vi "zs_example.vi"() -> ()   [LabVIEW 2014, in "Dialogue.lvlib" / "Dialogue.lvclass"]
uses:
  Dialogue.lvclass
  ctl/Point.ctl
panel:
  out "数值":dbl
  out "机器人语音指令数据簇数组(Voice)":T1(array[cluster])
  out "连接的字符串 2":string
  out "连接的字符串":string
  out "值(信号)":T2
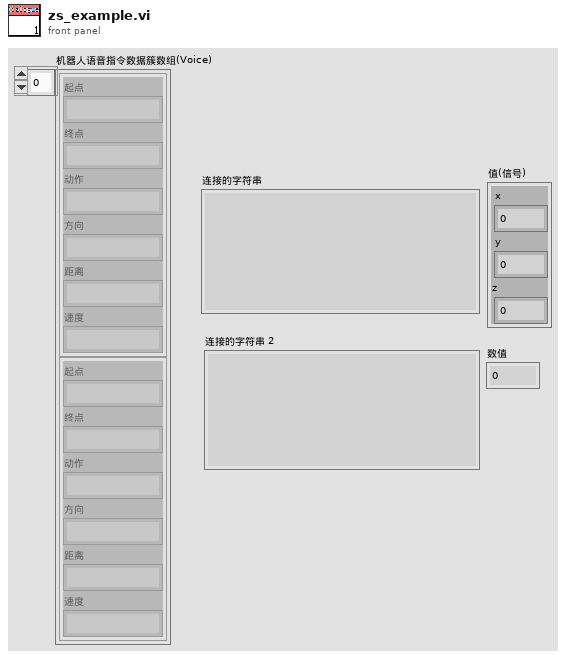
[diagram p1: front panel]
types:
  T1 = cluster{"起点":string, "终点":string, "动作":string, "方向":string, "距离":string, "速度":string}[]
  T2 = typedef "Point.ctl" = cluster{"x":dbl, "y":dbl, "z":dbl}
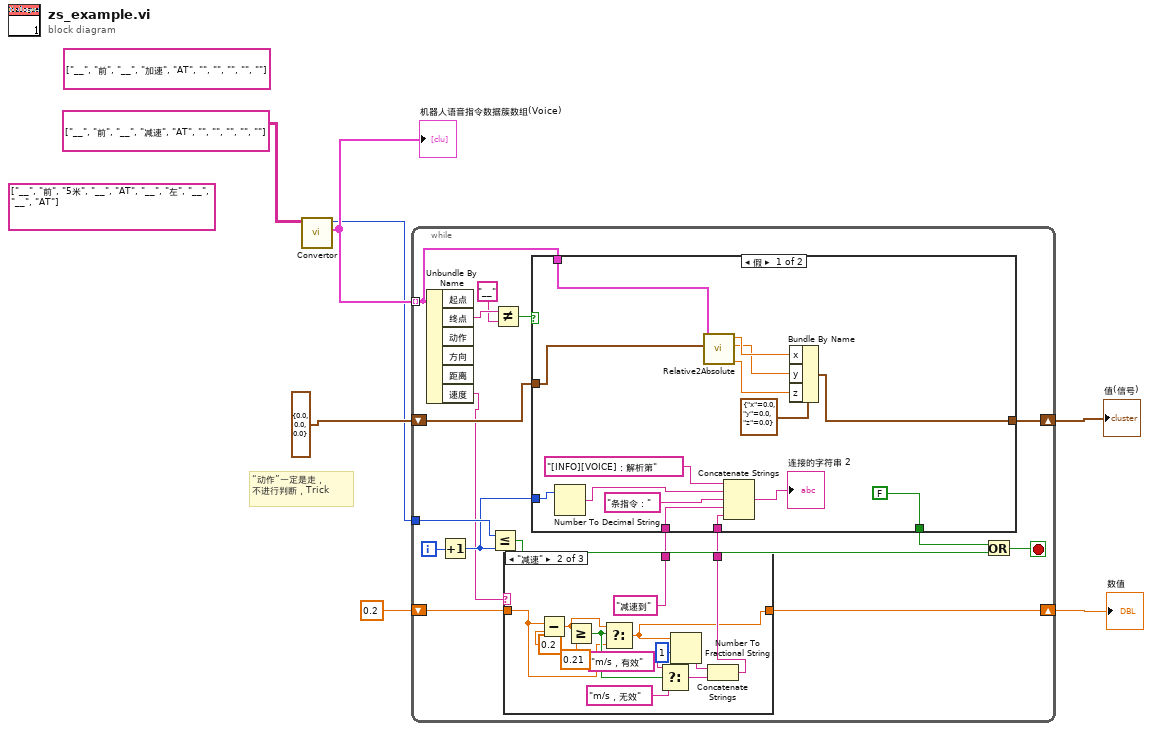
[diagram p0: block diagram]
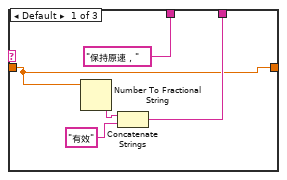
[diagram p2: hidden frame]
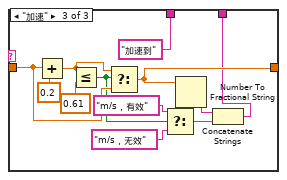
[diagram p3: hidden frame]
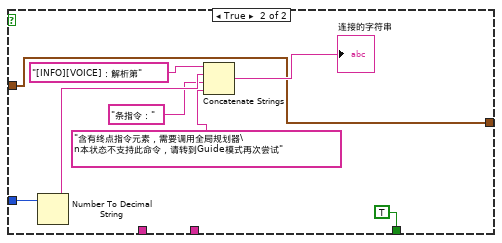
[diagram p4: hidden frame]
diagram:
  (unwired) string[][] [["__", "前", "__", "加速", "AT"], ["", "", "", "", ""]] ("格式化机器人指令 2")
  (unwired) string[][] [["__", "前", "5米", "__", "AT"], ["__", "左", "__", "__", "AT"]] ("格式化机器人指令 2")
  # "“动作”一定是走，\n不进行判断，Trick"
  n1 = call "Convertor.vi"("格式化机器人指令"=string[][] [["__", "前", "__", "减速", "AT"], ["", "", "", "", ""]] ("格式化机器人指令 2")) -> ("机器人语音指令数据簇数组(Voice)"=w5:T1, "命令个数"=w4:i32)  [unwired: 8 in, 1 out]
  "机器人语音指令数据簇数组(Voice)" <- w5
  n2 = while {
    tunnel: w5 -> [w21] mode=indexing
    shift-right: [w19] -> w7
    shift-left: T2 {"x"=0.0, "y"=0.0, "z"=0.0} ("值(信号)") -> [w18]
    tunnel: w4 -> [w16]
    shift-right: [w9] -> w1
    shift-left: 0.2 -> [w11]
    i -> [w20]
    stop <- w17 stop-if-true
    n3 = Unbundle By Name(w21) -> ("终点"=w24:string, "速度"=w12:string)  [unwired: 4 out]
    n4 = Increment(x=w20) -> (x+1=w15:i32)
    n5 = Less Or Equal?(x=w16, y=w15) -> (x <= y?=w14:bool)
    n6 = Not Equal?(x=w24, y="__") -> (x != y?=w22:bool)
    n7 = case shown="\"减速\"" w12 {
      tunnel: w11 -> [w25 w31 w50]
      tunnel: ["保持原速，" ("Event Text") "减速到" ("Event Text") "加速到" ("Event Text")] -> w10
      tunnel: [w25 w32 w45] -> w9
      tunnel: [w26 w33 w44] -> w8
      frame Default {
        n8 = Number To Fractional String(number=w25) -> (F-format string=w28:string)  [unwired: 3 in]
        n9 = Concatenate Strings(w28, "有效" ("Event Text")) -> (w26:string)
      }
      frame "减速" {
        n10 = Subtract(x=w31, y=0.2) -> (x-y=w40:dbl)
        n11 = Greater Or Equal?(x=w40, y=0.21) -> (x >= y?=w39:bool)
        n12 = Select(t=w40, s=w39, f=w31) -> (s? t:f=w32:dbl)
        n13 = Select(t="m/s，有效" ("Event Text"), s=w39, f="m/s，无效" ("Event Text")) -> (s? t:f=w36:string)
        n14 = Number To Fractional String(number=w32, precision (6)=i16 1 ("精度(6)")) -> (F-format string=w35:string)  [unwired: 2 in]
        n15 = Concatenate Strings(w35, w36) -> (w33:string)
      }
      frame "加速" {
        n16 = Add(x=w50, y=0.2) -> (x+y=w51:dbl)
        n17 = Less Or Equal?(x=w51, y=0.61) -> (x <= y?=w43:bool)
        n18 = Select(t=w51, s=w43, f=w50) -> (s? t:f=w45:dbl)
        n19 = Select(t="m/s，有效" ("Event Text"), s=w43, f="m/s，无效" ("Event Text")) -> (s? t:f=w47:string)
        n20 = Number To Fractional String(number=w45) -> (F-format string=w46:string)  [unwired: 3 in]
        n21 = Concatenate Strings(w46, w47) -> (w44:string)
      }
    }
    n22 = case shown="假" w22 {
      tunnel: [FALSE TRUE] -> w13
      tunnel: w21 -> [w63 _]
      tunnel: [w65 w70] -> w19
      tunnel: w18 -> [w64 w70]
      tunnel: w15 -> [w59 w76]
      tunnel: w10 -> [w56 _]
      tunnel: w8 -> [w55 _]
      frame False {
        n23 = Number To Decimal String(number=w59) -> (decimal integer string=w61:string)  [unwired: 1 in]
        n24 = call "Relative2Absolute.vi"("Ini_Pose"=w64, "机器人语音指令数据簇"=w63) -> ("Rot_deg"=w66:dbl, "y"=w67:dbl, "x"=w68:dbl)  [unwired: 7 in]
        n25 = Concatenate Strings("[INFO][VOICE]：解析第" ("Event Text"), w61, "条指令：" ("Event Text"), w56, w55) -> (→"连接的字符串 2":string)
        n26 = Bundle By Name(cluster=T2 {"x"=0.0, "y"=0.0, "z"=0.0} ("值(信号)"), "x"=w68, "y"=w67, "z"=w66) -> (w65:T2)
      }
      frame True {
        n27 = Number To Decimal String(number=w76) -> (decimal integer string=w74:string)  [unwired: 1 in]
        n28 = Concatenate Strings("[INFO][VOICE]：解析第" ("Event Text"), w74, "条指令：" ("Event Text"), "含有终点指令元素，需要调用全局规划器\n本状态不支持此命令，请转到Guide模式再次尝试" ("Event Text")) -> (→"连接的字符串":string)
      }
    }
    n29 = Or(x=w13, y=w14) -> (x .or. y?=w17:bool)
  }
  "值(信号)" <- w7
  "数值" <- w1
